vi "Close_GEA3_Serial.vi"(0 "session in":refnum<k35>, 11 "error in (no error)":errorcluster) -> (4 "session out":refnum<k35>, 15 "error out":errorcluster)   [LabVIEW 2021]
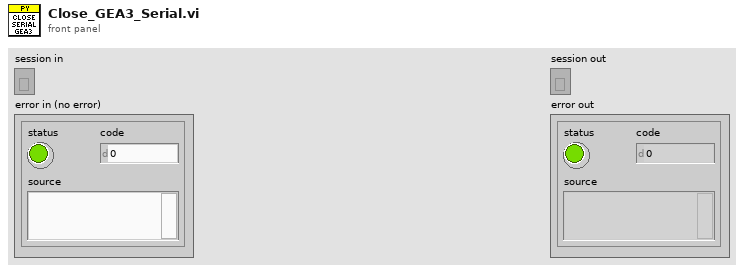
[diagram p1: front panel]
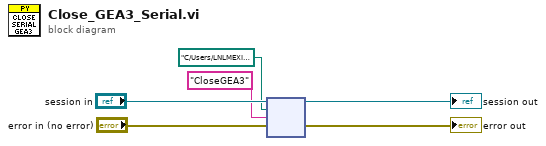
[diagram p0: block diagram]
diagram:
  n1 = node("session in", path "C:/Users/LNLMEXID/Desktop/GEA3 Python/Main.py" ("module path"), "CloseGEA3" ("function name"), "error in (no error)") -> (→"session out":refnum<k35>, →"error out":errorcluster)  [unwired: 2 in, 2 out]
